vi "Insert.vi"(8 "error in (no error)":errorcluster, 9 "Item":refnum<class>, 10 "Index":i32, 11 "List in":refnum<class "List.lvclass">) -> (0 "error out":errorcluster, 3 "List out":refnum<class "List.lvclass">)   [LabVIEW 2017, in "LapDog.Collections.v0.Lists.lvlib" / "List.lvclass"]
doc: "Inserts an item into the list at the location specified by Index, increasing the index of all items after the specified index by 1. If Index = -1 or Index = Count, the item is added to the end of the list. If Index < -1 or Index > Count, error 510301 is returned."
uses:
  List.lvclass
  List.lvclass/List.ctl
  ListImp/ListImp.lvclass
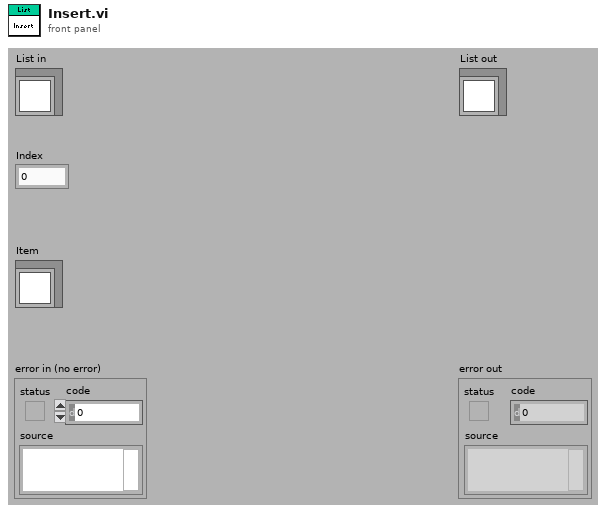
[diagram p1: front panel]
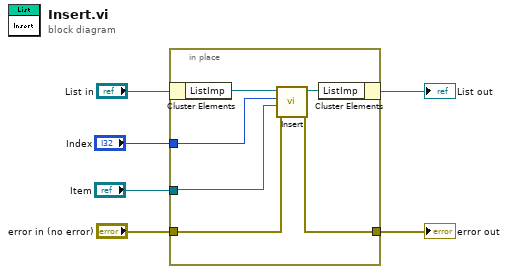
[diagram p0: block diagram]
diagram:
  n1 = in-place {
    in-place-border: "Item" -> [w10]
    in-place-border: "Index" -> [w9]
    in-place-border: "error in (no error)" -> [w8]
    in-place-border: [w7] -> w2
    n2 = in-place-cluster #1("List in") -> ("ListImp"=w12:refnum<class "ListImp.lvclass">)
    n3 = call-dynamic "Insert.vi"("error in (no error)"=w8, "Item"=w10, "Index"=w9, "ListImp in"=w12) -> ("error out"=w7:errorcluster, "ListImp out"=w11:refnum<class "ListImp.lvclass">)  [unwired: 6 in]
    n4 = in-place-cluster #1("ListImp"=w11) -> (→"List out":refnum<class "List.lvclass">)
  }
  "error out" <- w2
